vi "Main.vi"(8 "error in (no error)":errorcluster, 11 "Application in":refnum<class "SimonModel.lvclass">) -> (0 "error out":errorcluster, 3 "Application out":refnum<class "SimonModel.lvclass">)   [LabVIEW 2019, in "SimonModel.lvclass"]
doc: "Run this VI to lauch the State Machine."
uses:
  SimonModel.lvclass
  Context/Context.lvclass
panel:
  # "Run this VI to lauch the State Machine."
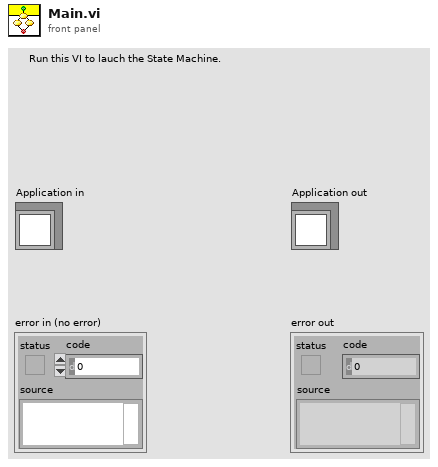
[diagram p1: front panel]
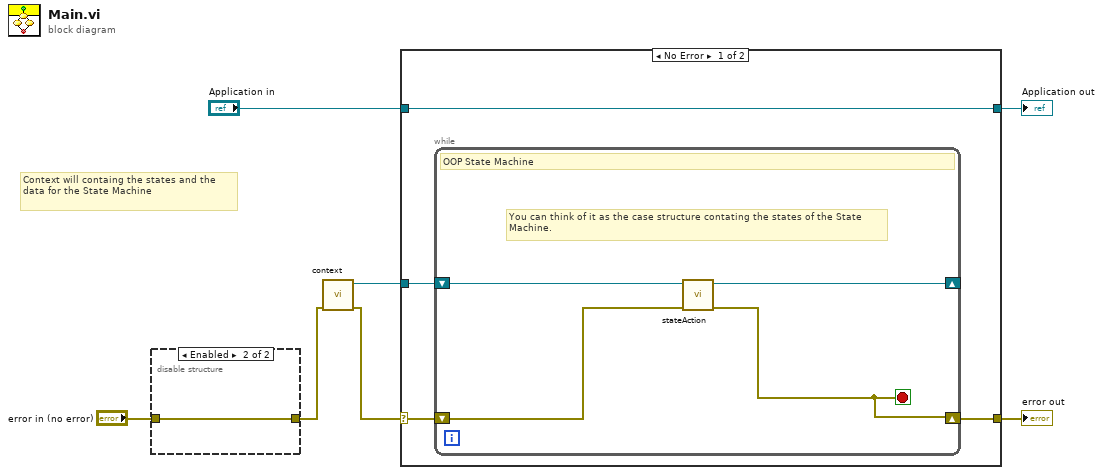
[diagram p0: block diagram]
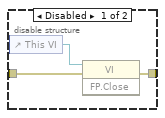
[diagram p2: hidden frame]
diagram:
  # "Context will containg the states and the\ndata for the State Machine"
  n1 = disable-structure shown="Enabled" {
    disable-tunnel: "error in (no error)" -> [w10 w11]
    disable-tunnel: [w9 w11] -> w2
    frame Disabled {
      n2 = control-ref of="This VI"() -> (w8:refnum<vi>)
      n3 = invoke class="VI" method="FP.Close"(reference=w8, error in=w10) -> (error out=w9:errorcluster)  [unwired: 1 in, 2 out]
    }
    frame Enabled {
    }
  }
  n4 = call "context.vi"("error in (no error)"=w2) -> ("error out"=w3:errorcluster, "Context Out"=w1:refnum<class "Context.lvclass">)  [unwired: 9 in]
  n5 = case shown="No Error" w3 {
    selector: w3 -> [w14 w21]
    tunnel: [w13 w21] -> w7
    tunnel: [w15 w20] -> w5
    tunnel: "Application in" -> [w15 w20]
    tunnel: w1 -> [w12 _]
    frame No Error {
      n6 = while {
        shift-right: [w16] -> w13
        shift-left: w14 -> [w19]
        shift-right: [w17] -> _
        shift-left: w12 -> [w18]
        stop <- w16 stop-if-true
        # "You can think of it as the case structure contating the states of the State\nMachine."
        # "OOP State Machine"
        n7 = call "stateAction.vi"("error in (no error)"=w19, "Context In"=w18) -> ("error out"=w16:errorcluster, "Context Out"=w17:refnum<class "Context.lvclass">)  [unwired: 8 in]
      }
    }
    frame Error {
    }
  }
  "error out" <- w7
  "Application out" <- w5
